vi "Generic Inst Names.vi"(4 "Analysis Info cluster":T1[](array[typedef]) {"Kurt_u" format="%_3g"; "u^4" format="%_3g"; "u^3" format="%_3g"; "Sd Error in Variance" format="%_3g"; "u^2" format="%_3g"; "Sd Error in Mean" format="%_3g"; "U" format="%_3g"; "Sync Delay Time (s)" format="%.4f"; "Total Meas Time (s)" format="%_5g"; "Skew_u" format="%_3g"; "% u'/U" format="%_3g"}) -> (1 "Analysis Info cluster out":T1[](array[typedef]) {"Kurt_u" format="%_3g"; "u^4" format="%_3g"; "u^3" format="%_3g"; "Sd Error in Variance" format="%_3g"; "u^2" format="%_3g"; "Sd Error in Mean" format="%_3g"; "U" format="%_3g"; "Sync Delay Time (s)" format="%.4f"; "Total Meas Time (s)" format="%_5g"; "Skew_u" format="%_3g"; "% u'/U" format="%_3g"})   [LabVIEW 2022 SP3]
uses:
  Globals/Meas_global.vi
  Controls/Inst_type.ctl
  Controls/Instrument_Array.ctl
  Controls/Analysis_info_cluster.ctl
  Controls/channelState.ctl
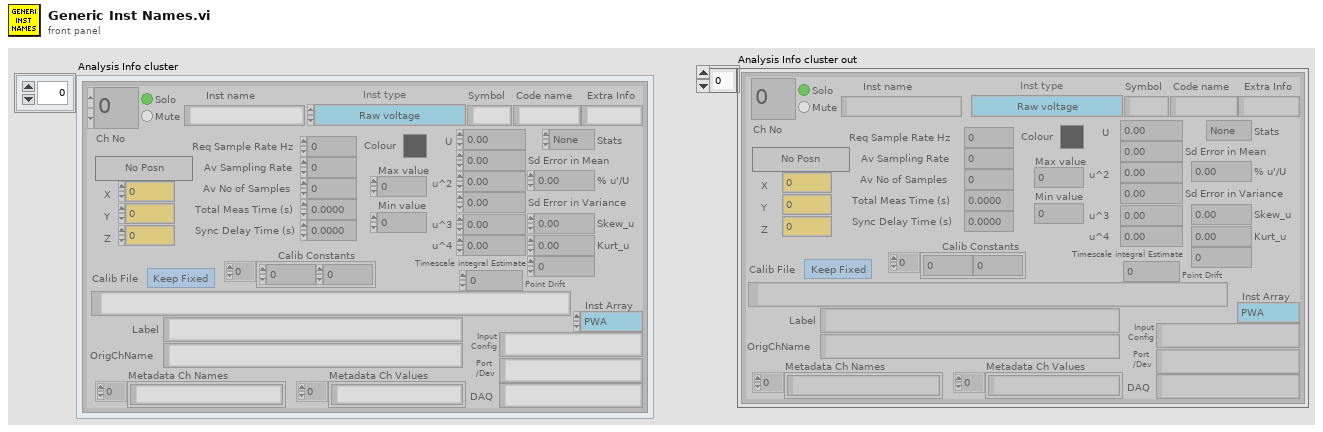
[diagram p1: front panel]
types:
  T1 = typedef "Analysis_info_cluster.ctl" = cluster{"Colour":u32, "Inst type":T2, "Inst name":string, "Symbol":string, "Code name":string, "Extra Info":string, "Inst Array":T3, "U":dbl, "u^2":dbl, "u^3":dbl, "u^4":dbl, "Skew_u":dbl, "Kurt_u":dbl, "Sd Error in Mean":dbl, "% u'/U":dbl, "X":dbl, "Y":dbl, "Z":dbl, "Timescale integral Estimate":dbl, "Sd Error in Variance":dbl, "Calib File":path, "Calib Constants":dbl[], "Output Position":bool, "Stats":enum16{"None", "Basic", "Full"}, "Av Sampling Rate":dbl, "Av No of Samples":dbl, "Total Meas Time (s)":dbl, "OrigChName":string, "Max value":dbl, "Min value":dbl, "Req Sample Rate Hz":dbl, "Sync Delay Time (s)":dbl, "Ch No":i16, "Device":string, "Use Latest Calib":bool, "Port":string, "Metadata Ch Names":string[], "Metadata Ch Values":string[], "Label":string, "chState":T4, "Point Drift":dbl, "inputConfig":string}
  T2 = typedef "Inst_type.ctl" = enum16{"Raw voltage", "Raw with zero offsetting", "Propeller anemometer", "Pressure Transducer", "Pitot-static tube", "Hot wire", "Cross wire 1", "Cross wire 2", "Generic Linear", "Generic Polynomial", "Generic BackPoly", "Fast FID", "Thermocouple", "Cold wire", "Pulsed Wire", "LDA Vel", "LDA Tran time", "LDA Arr time", "Microphone"}
  T3 = typedef "Instrument_Array.ctl" = enum16{"PWA", "LDA", "Analogue"}
  T4 = typedef "channelState.ctl" = enum32{"No Selection", "Solo", "Mute"}
  T5 = typedef "Initial Info Cluster.ctl" = cluster{"Metadata Ch Names":string[], "Metadata Ch Values":string[]}
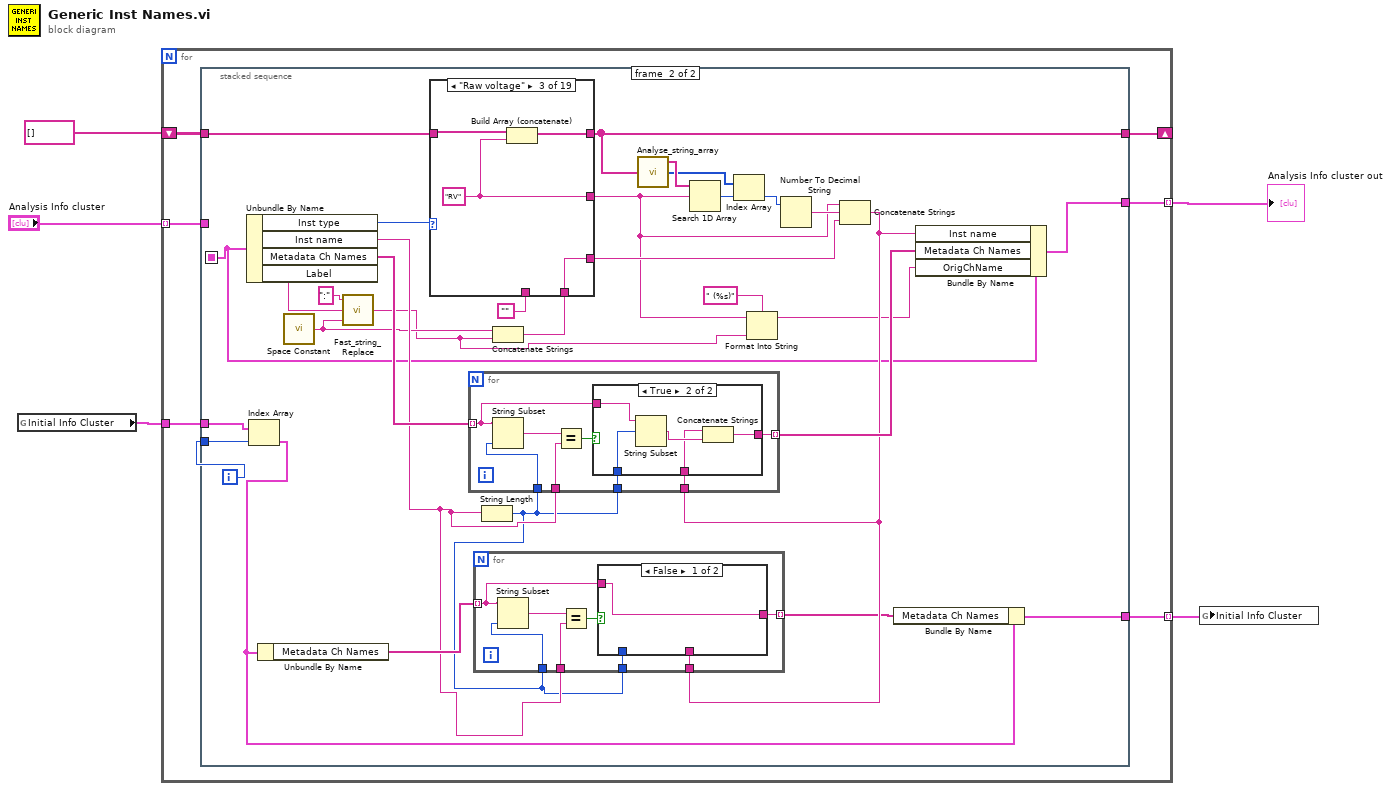
[diagram p0: block diagram]
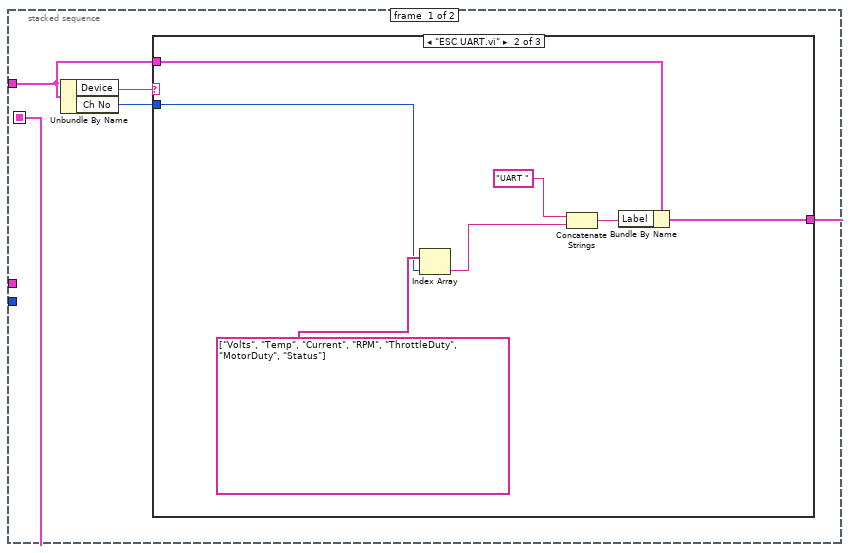
[diagram p2: hidden frame]
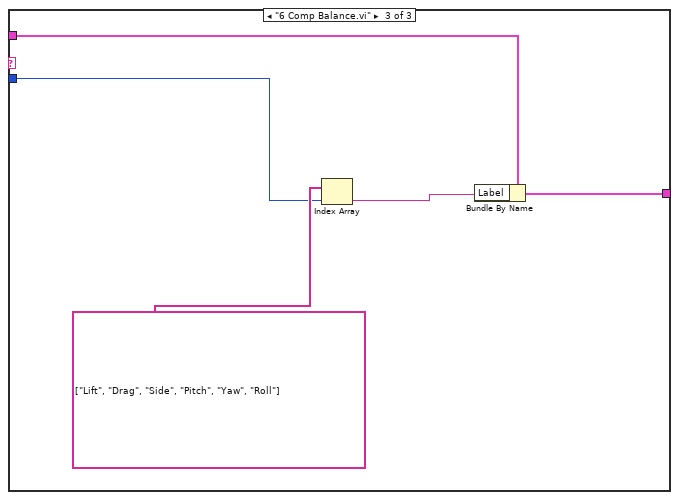
[diagram p4: hidden frame]
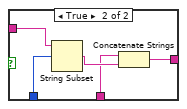
[diagram p5: hidden frame]
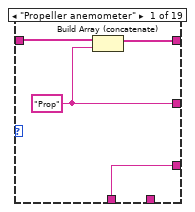
[diagram p7: hidden frame]
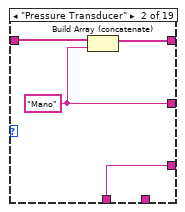
[diagram p8: hidden frame]
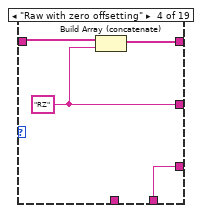
[diagram p9: hidden frame]
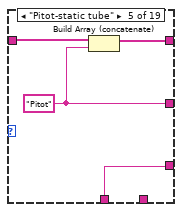
[diagram p10: hidden frame]
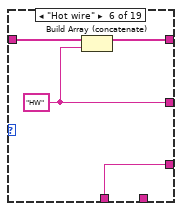
[diagram p11: hidden frame]
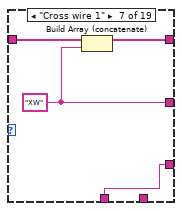
[diagram p12: hidden frame]
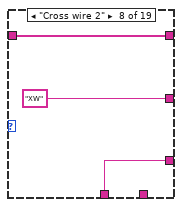
[diagram p13: hidden frame]
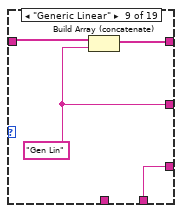
[diagram p14: hidden frame]
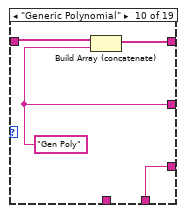
[diagram p15: hidden frame]
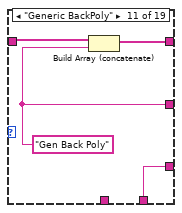
[diagram p16: hidden frame]
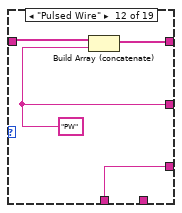
[diagram p17: hidden frame]
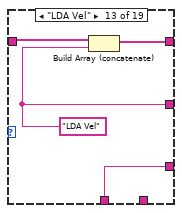
[diagram p18: hidden frame]
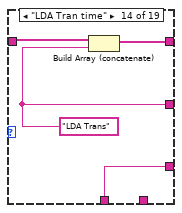
[diagram p19: hidden frame]
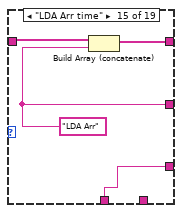
[diagram p20: hidden frame]
diagram:
  n1 = global read "Meas_global.vi" "Initial Info Cluster"() -> (w2:T5[])
  n2 = for {
    shift-right: [w11] -> _
    shift-left: string[] [] -> [w12]
    tunnel: "Analysis Info cluster" -> [w10] mode=indexing
    tunnel: [w9] -> w3 mode=indexing
    tunnel: w2 -> [w7]
    tunnel: [w8] -> w1 mode=indexing
    i -> [w6]
    n3 = stacked-sequence {
      seq-local: [w13 _] -> [_ w38]
      tunnel: w12 -> [_ w56]
      tunnel: [_ w55] -> w11
      tunnel: w10 -> [w14 _]
      tunnel: [_ w37] -> w9
      tunnel: [_ w45] -> w8
      tunnel: w7 -> [_ w44]
      tunnel: w6 -> [_ w43]
      frame #0 {
        n4 = Unbundle By Name(w14) -> ("Device"=w16:string, "Ch No"=w15:i16)
        n5 = case shown="\"ESC UART.vi\"" w16 {
          tunnel: w14 -> [w17 w24 w29]
          tunnel: [w17 w23 w28] -> w13
          tunnel: w15 -> [_ w21 w26]
          frame Default {
          }
          frame "ESC UART.vi" {
            n6 = Index Array(array=string[] ["Volts", "Temp", "Current", "RPM", "ThrottleDuty", "MotorDuty", "Status"], index=w21) -> (element=w19:string)
            n7 = Concatenate Strings("UART " ("string"), w19) -> (w20:string)
            n8 = Bundle By Name(cluster=w24, "Label"=w20) -> (w23:T1)
          }
          frame "6 Comp Balance.vi" {
            n9 = Index Array(array=string[] ["Lift", "Drag", "Side", "Pitch", "Yaw", "Roll"], index=w26) -> (element=w25:string)
            n10 = Bundle By Name(cluster=w29, "Label"=w25) -> (w28:T1)
          }
        }
      }
      frame #1 {
        n11 = Unbundle By Name(w38) -> ("Inst type"=w57:T2, "Inst name"=w49:string, "Metadata Ch Names"=w52:string[], "Label"=w36:string)
        n12 = Index Array(array=w44, index=w43) -> (element=w42:T5)
        n13 = Unbundle By Name(w42) -> ("Metadata Ch Names"=w50:string[])
        n14 = call <vilib>:"Space Constant.vi"() -> ("String"=w34:string)
        n15 = call "Fast_string_Replace.vi"("Replace match with:"=w34, "Input String"=w36, "matchThis"=":") -> ("Output String"=w32:string)  [unwired: 1 in, 1 out]
        n16 = String Length(string=w49) -> (length=w48:i32)
        n17 = Concatenate Strings(w34, w32) -> (w39:string)
        n18 = case shown="\"Raw voltage\"" w57 {
          tunnel: [w91 w95 w98 w102 w106 w110 w114 "XW" w121 w125 w129 w133 w137 w141 w145 w149 w154 w157 w161] -> w33
          tunnel: w56 -> [w92 w96 w100 w104 w108 w112 w116 w118 w123 w127 w131 w135 w139 w143 w147 w151 w155 w159 w163]
          tunnel: [w90 w94 w99 w103 w107 w111 w115 w118 w122 w126 w130 w134 w138 w142 w146 w150 w153 w158 w162] -> w55
          tunnel: [w89 w93 w97 w101 w105 w109 w113 w117 w120 w124 w128 w132 w136 w140 w144 w148 w152 w156 w160] -> w40
          tunnel: "" -> [w89 w93 _ _ w105 w109 w113 w117 _ _ _ w132 w136 w140 w144 w148 w152 w156 w160]
          tunnel: w39 -> [_ _ w97 w101 _ _ _ _ w120 w124 w128 _ _ _ _ _ _ _ _]
          frame "Propeller anemometer" {
            w91 = "Prop"
            n19 = Build Array (concatenate)(w92, w91) -> (w90:string[])
          }
          frame "Pressure Transducer" {
            w95 = "Mano"
            n20 = Build Array (concatenate)(w96, w95) -> (w94:string[])
          }
          frame "Raw voltage" {
            w98 = "RV"
            n21 = Build Array (concatenate)(w100, w98) -> (w99:string[])
          }
          frame "Raw with zero offsetting" {
            w102 = "RZ"
            n22 = Build Array (concatenate)(w104, w102) -> (w103:string[])
          }
          frame "Pitot-static tube" {
            w106 = "Pitot"
            n23 = Build Array (concatenate)(w108, w106) -> (w107:string[])
          }
          frame "Hot wire" {
            w110 = "HW"
            n24 = Build Array (concatenate)(w112, w110) -> (w111:string[])
          }
          frame "Cross wire 1" {
            w114 = "XW"
            n25 = Build Array (concatenate)(w116, w114) -> (w115:string[])
          }
          frame "Cross wire 2" {
          }
          frame "Generic Linear" {
            w121 = "Gen Lin"
            n26 = Build Array (concatenate)(w123, w121) -> (w122:string[])
          }
          frame "Generic Polynomial" {
            w125 = "Gen Poly"
            n27 = Build Array (concatenate)(w127, w125) -> (w126:string[])
          }
          frame "Generic BackPoly" {
            w129 = "Gen Back Poly"
            n28 = Build Array (concatenate)(w131, w129) -> (w130:string[])
          }
          frame "Pulsed Wire" {
            w133 = "PW"
            n29 = Build Array (concatenate)(w135, w133) -> (w134:string[])
          }
          frame "LDA Vel" {
            w137 = "LDA Vel"
            n30 = Build Array (concatenate)(w139, w137) -> (w138:string[])
          }
          frame "LDA Tran time" {
            w141 = "LDA Trans"
            n31 = Build Array (concatenate)(w143, w141) -> (w142:string[])
          }
          frame "LDA Arr time" {
            w145 = "LDA Arr"
            n32 = Build Array (concatenate)(w147, w145) -> (w146:string[])
          }
          frame "Microphone" {
            w149 = "Mic"
            n33 = Build Array (concatenate)(w151, w149) -> (w150:string[])
          }
          frame "Fast FID" {
            w154 = "FF"
            n34 = Build Array (concatenate)(w155, w154) -> (w153:string[])
          }
          frame "Thermocouple" {
            w157 = "T"
            n35 = Build Array (concatenate)(w159, w157) -> (w158:string[])
          }
          frame "Cold wire" {
            w161 = "CW"
            n36 = Build Array (concatenate)(w163, w161) -> (w162:string[])
          }
        }
        n37 = call "Analyse_string_array.vi"("String array"=w55) -> ("Unique strings"=w60:string[], "Frequency"=w58:i32[])  [unwired: 1 out]
        n38 = Search 1D Array(1D array=w60, element=w33) -> (index of element=w59:i32)  [unwired: 1 out]
        n39 = Index Array(array=w58, index=w59) -> (element=w54:i32)
        n40 = Format Into String(format string=" (%s)", initial string=w33, w32) -> (resulting string=w30:string)  [unwired: 1 in, 1 out]
        n41 = Number To Decimal String(number=w54) -> (decimal integer string=w53:string)  [unwired: 1 out]
        n42 = Concatenate Strings(w33, w53, w40) -> (w47:string)
        n43 = for {
          tunnel: w52 -> [w78] mode=indexing
          tunnel: w48 -> [w82]
          tunnel: w49 -> [w80]
          tunnel: w48 -> [w79]
          tunnel: w47 -> [w77]
          tunnel: [w76] -> w51 mode=indexing
          n44 = String Subset(string=w78, length (rest)=w82) -> (substring=w81:string)  [unwired: 1 in]
          n45 = Equal?(x=w81, y=w80) -> (x = y?=w75:bool)
          n46 = case shown="True" w75 {
            tunnel: w79 -> [_ w88]
            tunnel: w78 -> [w83 w87]
            tunnel: w77 -> [_ w85]
            tunnel: [w83 w84] -> w76
            frame False {
            }
            frame True {
              n47 = String Subset(string=w87, offset (0)=w88) -> (substring=w86:string)  [unwired: 1 in]
              n48 = Concatenate Strings(w85, w86) -> (w84:string)
            }
          }
        }
        n49 = for {
          tunnel: w50 -> [w64] mode=indexing
          tunnel: w48 -> [w68]
          tunnel: w49 -> [w66]
          tunnel: w48 -> [w65]
          tunnel: w47 -> [w63]
          tunnel: [w62] -> w46 mode=indexing
          n50 = String Subset(string=w64, length (rest)=w68) -> (substring=w67:string)  [unwired: 1 in]
          n51 = Equal?(x=w67, y=w66) -> (x = y?=w61:bool)
          n52 = case shown="False" w61 {
            tunnel: w65 -> [_ w74]
            tunnel: w64 -> [w69 w73]
            tunnel: w63 -> [_ w71]
            tunnel: [w69 w70] -> w62
            frame False {
            }
            frame True {
              n53 = String Subset(string=w73, offset (0)=w74) -> (substring=w72:string)  [unwired: 1 in]
              n54 = Concatenate Strings(w71, w72) -> (w70:string)
            }
          }
        }
        n55 = Bundle By Name(cluster=w42, "Metadata Ch Names"=w46) -> (w45:T5)
        n56 = Bundle By Name(cluster=w38, "Inst name"=w47, "Metadata Ch Names"=w51, "OrigChName"=w30) -> (w37:T1)
      }
    }
  }
  "Analysis Info cluster out" <- w3
  n57 = global write "Meas_global.vi" "Initial Info Cluster"(w1) -> ()
